vi "Save.vi"(8 "error in":errorcluster, 10 "file path":path, 11 "repository in":refnum<class "CustomDeviceRepo.lvclass">) -> (0 "error out":errorcluster, 3 "repository out":refnum<class "CustomDeviceRepo.lvclass">)   [LabVIEW 2019, in "CustomDeviceRepo.lvclass"]
doc: "Stores repo information to file. It could save in multiple files or formats at the same time. File versioning is suggested."
uses:
  CustomDeviceRepo.lvclass
  NationalInstruments.VeriStand.XMLReader
  CustomDeviceRepo.lvclass/CustomDeviceRepo.ctl
  VeriStand Custom Device XML Parser.lvlib
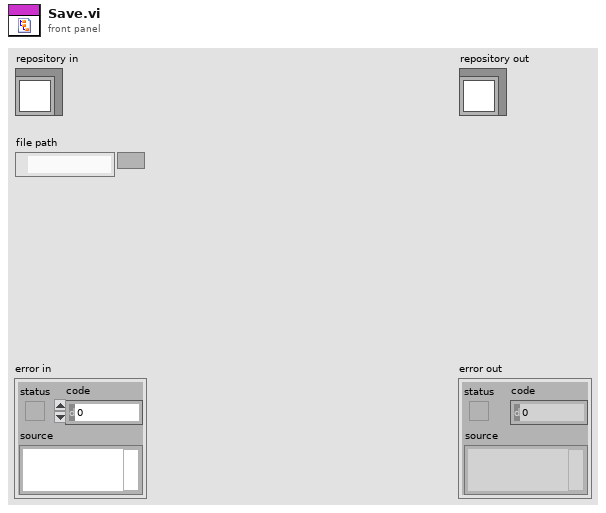
[diagram p1: front panel]
types:
  T1 = typedef "VeriStand Custom Device XML Parser.lvlib/Main Custom Device Properties.ctl" = cluster{"CD Name":string, "Version":string, "Max Occurrences":i32, "Device Type":enum16{"Asynchronous", "Inline HW Interface", "Inline Model Interface", "Inline Timing and Sync", "Asynchronous Timing and Sync"}, "Main Page GUID":string}
  T2 = typedef "VeriStand Custom Device XML Parser.lvlib/Initialization VI Properties.ctl" = cluster{"Execution":T3, "Path":T4, "Type":enum16{"Action", "VI"}, "Position":enum16{"centered", "mouse pointer"}}
  T3 = typedef "VeriStand Custom Device XML Parser.lvlib/Execution Types.ctl" = enum16{"silent", "modal", "floating", "default"}
  T4 = typedef "VeriStand Custom Device XML Parser.lvlib/Path Cluster.ctl" = cluster{"Path":path, "Path Type":enum16{"Absolute", "To Base", "To Common Doc Dir", "To Application Data Dir"}}
  T5 = typedef "VeriStand Custom Device XML Parser.lvlib/Timing Source Properties.ctl" = cluster{"Has Timing Source Capability":bool, "Source Distribution":T6}
  T6 = typedef "VeriStand Custom Device XML Parser.lvlib/Timing Source Source Distribution Properties.ctl" = cluster{"Supported Target":T7, "Source":T4, "Real Time System Destination":string, "Version":string}[]
  T7 = typedef "VeriStand Custom Device XML Parser.lvlib/Supported Targets.ctl" = enum16{"All", "Pharlap", "VxWorks", "Windows", "Linux_32_ARM", "Linux_x64", "PharlapWindows", "PharlapVxWorks", "VxWorksWindows"}
  T8 = typedef "VeriStand Custom Device XML Parser.lvlib/Custom Device Source Distribution Properties.ctl" = cluster{"Source":T4, "Real Time System Destination":string, "Supported Target":T7}[]
  T9 = typedef "VeriStand Custom Device XML Parser.lvlib/Page Properties.ctl" = cluster{"Name":string, "Disallow Renaming":bool, "Delete Protection":bool, "Exlcude from Alphabetical order":bool, "Allow Multi-Selection":bool, "GUID":string, "Parent GUIDs":string[], "Glyph":T4, "Inactive Glyph":T4, "Broken Glyph":T4, "Item to Launch":T4, "Additional Information":string, "Copy":enum16{"copy", "disabled"}, "Paste":enum16{"Create", "CreatIfNotExists_GUID", "CreatIfNotExists_Name", "Replace", "Dialog"}, "Help":T10}
  T10 = typedef "VeriStand Custom Device XML Parser.lvlib/Help File Properties.ctl" = cluster{"Item to Launch":T4, "Section":string, "File Type":enum16{"chm", "other"}}
  T11 = typedef "VeriStand Custom Device XML Parser.lvlib/ActionVIs Properties.ctl" = cluster{"Action VI On Delete":T4, "Action VI On Load":T4, "Action VI On Paste":T4, "Action VI On Target Type Change":T4, "Action VI On Delete Request":T4, "Action VI On Compile":T4, "Action VI On System Shutdown":T4, "Action VI On Save":T4, "Action VI On Download":T4}
  T12 = typedef "VeriStand Custom Device XML Parser.lvlib/ButtonLists Properties.ctl" = cluster{"ID":string, "Glyph":T4, "Button Type":T13, "Referenced GUID":string, "Button Text":string, "Caption":string, "Tip Strip":string, "Documentation":string, "Dependency":T14}
  T13 = typedef "VeriStand Custom Device XML Parser.lvlib/Button Type.ctl" = enum16{"Action", "Dialog", "Page", "Notification", "Separator"}
  T14 = typedef "VeriStand Custom Device XML Parser.lvlib/Dependency Properties.ctl" = cluster{"File Path Control":path, "Path Type":enum16{"Absolute", "To Base", "To Common Doc Dir", "To Application Data Dir"}, "Behavior":enum16{"Static", "Dynamic"}}
  T15 = typedef "VeriStand Custom Device XML Parser.lvlib/RunTimeMenus Properties.ctl" = cluster{"GUID":string, "Execution":T3, "MinNrOfChilds":u32, "Name":string, "Item to Launch":T4, "Dependency":T14, "Custom Population":T4, "Menu Item Type":enum16{"Action", "VI", "Separator", "Custom"}, "Behavior":enum16{"Nothing", "Open Front Panel"}, "Position":enum16{"Centered", "Mouse Pointer"}}
  T16 = cluster{"General Page Properties":T9, "ActionVIs Properties":T11, "Button List Properties":T12[], "RunTime Menus Properties":T15[]}[]
  T17 = typedef "VeriStand Custom Device XML Parser.lvlib/Dependencies Properties.ctl" = cluster{"ForceDownload":bool, "RealTimeSystemDestination":string, "Path Properties":T4, "Supported Target":T7, "Version":string, "SupportedTargetSpecified":bool}
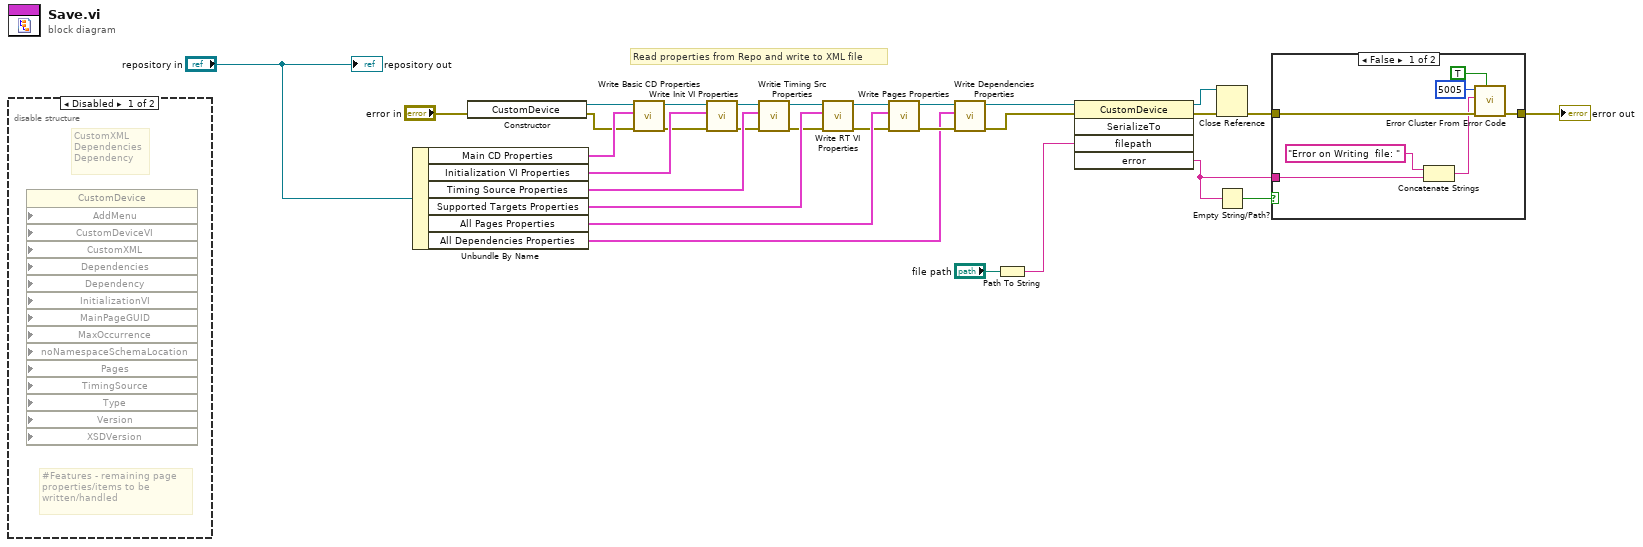
[diagram p0: block diagram]
diagram:
  # "Read properties from Repo and write to XML file"
  n1 = disable-structure shown="Disabled" {
    frame Disabled {
      # "#Features - remaining page\nproperties/items to be\nwritten/handled"
      # "CustomXML\nDependencies\nDependency"
      n2 = property class="CustomDevice" props=["AddMenu", "CustomDeviceVI", "CustomXML", "Dependencies", "Dependency", "InitializationVI", "MainPageGUID", "MaxOccurrence", "noNamespaceSchemaLocation", "Pages", "TimingSource", "Type", "Version", "XSDVersion"]() -> ()  [unwired: 16 in, 2 out]
    }
    frame Enabled {
    }
  }
  n3 = Unbundle By Name("repository in") -> ("Main CD Properties"=w26:T1, "Initialization VI Properties"=w23:T2, "Timing Source Properties"=w20:T5, "Supported Targets Properties"=w17:T8, "All Pages Properties"=w14:T16, "All Dependencies Properties"=w1:T17[])
  n4 = constructor class="CustomDevice"(error in="error in") -> (reference out=w27:refnum<k24>, error out=w25:errorcluster)  [unwired: 2 in, 1 out]
  n5 = call "Write Basic CD Properties.vi"("Error In"=w25, "Main CD Properties"=w26, "Custom Device .NET Ref In"=w27) -> ("Error Out"=w22:errorcluster, "Custom Device .NET Ref Out"=w24:refnum<k24>)  [unwired: 7 in]
  n6 = call "Write Init VI Properties.vi"("Error In"=w22, "Initialization VI Properties"=w23, "Custom Device .NET Ref In"=w24) -> ("Error Out"=w19:errorcluster, "Custom Device .NET Ref Out"=w21:refnum<k24>)  [unwired: 7 in]
  n7 = call "Writie Timing Src Properties.vi"("Error In"=w19, "Timing Source Properties"=w20, "Custom Device .NET Ref In"=w21) -> ("Error Out"=w16:errorcluster, "Custom Device .NET Ref Out"=w18:refnum<k24>)  [unwired: 7 in]
  n8 = call "Write RT VI Properties.vi"("Error In"=w16, "Supported Targets Properties"=w17, "Custom Device .NET Ref In"=w18) -> ("Error Out"=w13:errorcluster, "Custom Device .NET Ref Out"=w15:refnum<k24>)  [unwired: 7 in]
  n9 = call "Write Pages Properties.vi"("Error In"=w13, "All Pages Properties"=w14, "Custom Device .NET Ref In"=w15) -> ("Error Out"=w2:errorcluster, "Custom Device .NET Ref Out"=w5:refnum<k24>)  [unwired: 7 in]
  n10 = call "Write Dependencies Properties.vi"("Error In"=w2, "All Dependencies Properties"=w1, "Custom Device .NET Ref In"=w5) -> ("Error Out"=w3:errorcluster, "Custom Device .NET Ref Out"=w4:refnum<k24>)  [unwired: 7 in]
  n11 = Path To String(path="file path") -> (string=w11:string)
  n12 = invoke class="CustomDevice" method="SerializeTo"(reference=w4, error in=w3, "filepath"=w11) -> (reference out=w8:refnum<k24>, error out=w7:errorcluster, "error"=w9:string)  [unwired: 2 in, 2 out]
  n13 = Close Reference(reference=w8, error in (no error)=w7) -> (error out=w6:errorcluster)
  n14 = Empty String/Path?(string/path=w9) -> (empty?=w10:bool)
  n15 = case shown="False" w10 {
    tunnel: w9 -> [w36 _]
    tunnel: w6 -> [w35 w38]
    tunnel: [w32 w38] -> w28
    frame False {
      n16 = Concatenate Strings("Error on Writing  file: " ("string"), w36) -> (w33:string)
      n17 = call <vilib>:"Error Cluster From Error Code.vi"("show call chain? (False)"=TRUE, "error in (no error)"=w35, "error message (\"\")"=w33, "error code (0)"=5005) -> ("error out"=w32:errorcluster)  [unwired: 5 in]
    }
    frame True {
    }
  }
  "error out" <- w28
  "repository out" <- "repository in"
